vi "创建加工类.vi"(8 "error in (no error)":errorcluster caption="错误输入（无错误）", 11 "加工方法":T1) -> (0 "error out":errorcluster caption="错误输出", 3 "加工类（抽象）.lvclass":refnum<class "加工类（抽象）.lvclass">)   [LabVIEW 2011, in "简单加工类工厂.lvclass"]
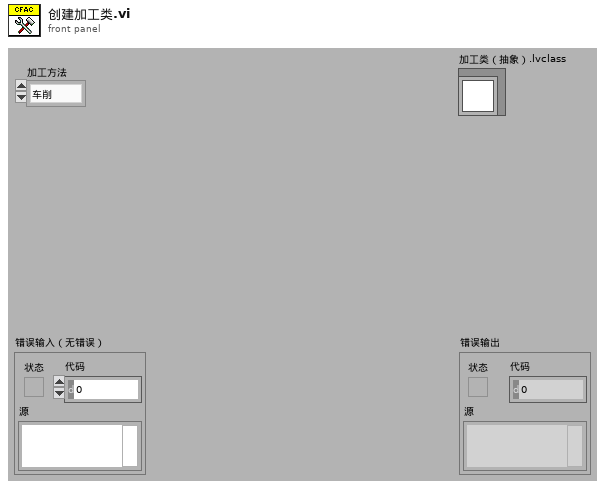
[diagram p1: front panel]
types:
  T1 = typedef "简单加工类工厂.lvclass/加工方法.ctl" = enum16{"车削", "铣削", "钻削"}
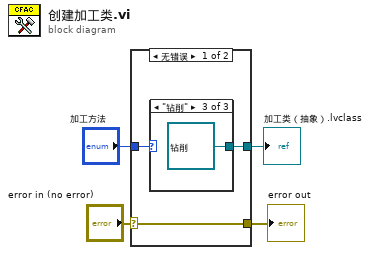
[diagram p0: block diagram]
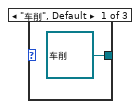
[diagram p2: hidden frame]
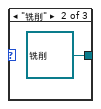
[diagram p3: hidden frame]
diagram:
  n1 = case shown="无错误" "error in (no error)" {
    selector: "error in (no error)" -> [w7 w11]
    tunnel: [w7 w11] -> w3
    tunnel: "加工方法" -> [w6 _]
    tunnel: [w5 _] -> w1
    frame No Error {
      n2 = case shown="\"钻削\"" w6 {
        tunnel: [refnum<class "车削.lvclass"> refnum ("车削.lvclass") refnum<class "铣削.lvclass"> refnum ("铣削.lvclass") refnum<class "钻削.lvclass"> refnum ("钻削.lvclass")] -> w5
        frame "车削", Default {
        }
        frame "铣削" {
        }
        frame "钻削" {
        }
      }
    }
    frame Error {
    }
  }
  "error out" <- w3
  "加工类（抽象）.lvclass" <- w1
